vi "Create (PNG with Alpha).vi"(8 "error in (no error)":errorcluster) -> (0 "error out":errorcluster, 3 "Image to File-Buffer Encoder":refnum<class "Image to File-Buffer Encoder.lvclass">)   [LabVIEW 2020, in "image.lvlib" / "Image to File-Buffer Encoder.lvclass"]
uses:
  Image to File-Buffer Encoder.lvclass
  Image to File-Buffer Encoder.lvclass/Image to File-Buffer Encoder.ctl
  6664653f-8b96-48f7-b608-248a9502c1d9.vi
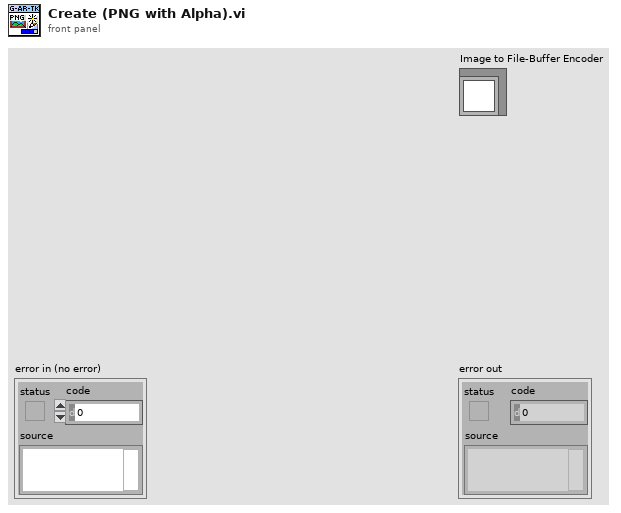
[diagram p1: front panel]
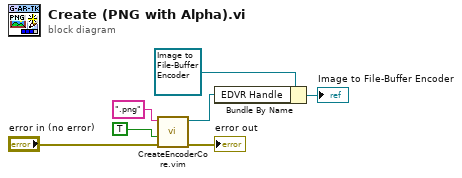
[diagram p0: block diagram]
diagram:
  n1 = call "CreateEncoderCore.vim"("error in (no error)"="error in (no error)", "SaveAlpha"=TRUE, "Extension"=".png") -> ("error out"=→"error out":errorcluster, "EDVR Handle"=w3:refnum<data-value>)  [unwired: 7 in]
  n2 = Bundle By Name(cluster=refnum<class "Image to File-Buffer Encoder.lvclass"> refnum ("Image to File-Buffer Encoder out"), "EDVR Handle"=w3) -> (→"Image to File-Buffer Encoder":refnum<class "Image to File-Buffer Encoder.lvclass">)
